vi "速度轉電壓.vi"(1 "Speed (0.1mm/s)":dbl) -> (0 "Voltage\nOutput":dbl)   [LabVIEW 2019]
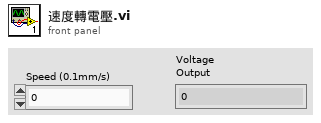
[diagram p1: front panel]
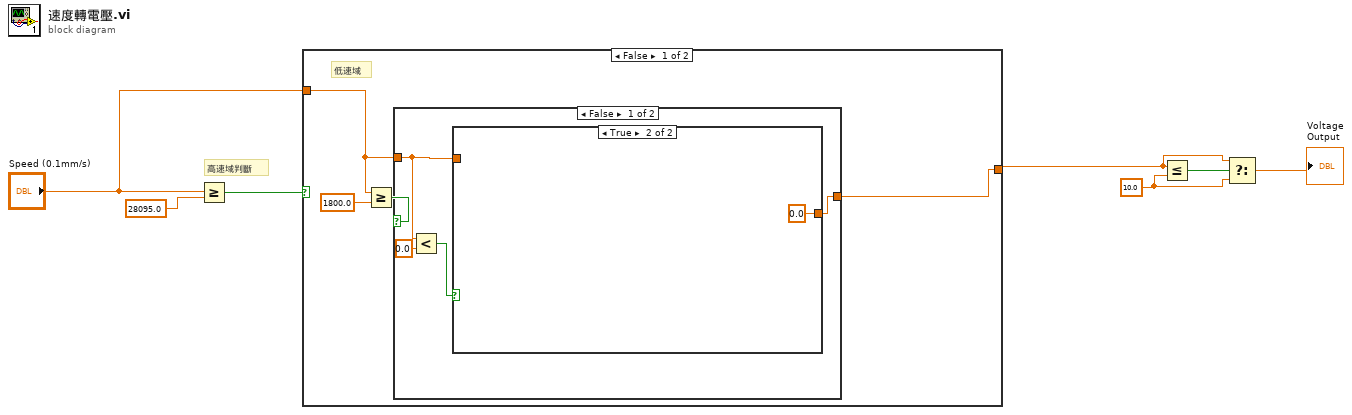
[diagram p0: block diagram]
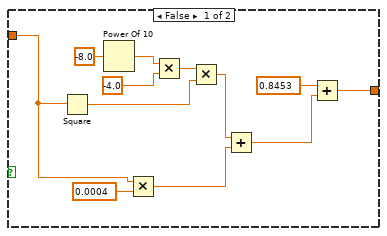
[diagram p2: hidden frame]
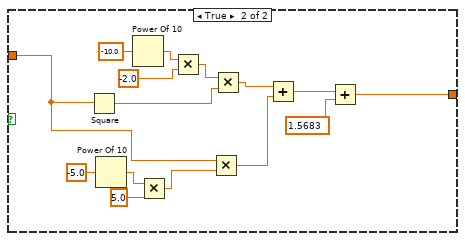
[diagram p3: hidden frame]
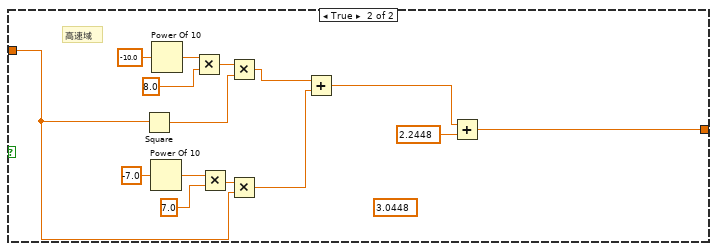
[diagram p4: hidden frame]
diagram:
  w2 = 10.0 ("y")
  # "高速域判斷"
  n1 = Greater Or Equal?(x="Speed (0.1mm/s)", y=28095.0) -> (x >= y?=w6:bool)
  n2 = case shown="False" w6 {
    tunnel: "Speed (0.1mm/s)" -> [w9 w48]
    tunnel: [w8 w58] -> w3
    frame False {
      # "低速域"
      n3 = Greater Or Equal?(x=w9, y=1800.0) -> (x >= y?=w10:bool)
      n4 = case shown="False" w10 {
        tunnel: w9 -> [w13 w34]
        tunnel: [w15 w30] -> w8
        frame False {
          n5 = Less?(x=w13, y=0.0) -> (x < y?=w14:bool)
          n6 = case shown="True" w14 {
            tunnel: [w17 0.0] -> w15
            tunnel: w13 -> [w16 _]
            frame False {
              n7 = Square(x=w16) -> (x^2=w27:dbl)
              n8 = Power Of 10(x=-8.0) -> (10^x=w22:dbl)
              n9 = Multiply(x=w16, y=0.0004) -> (x*y=w24:dbl)
              n10 = Multiply(x=w22, y=-4.0) -> (x*y=w26:dbl)
              n11 = Multiply(x=w26, y=w27) -> (x*y=w25:dbl)
              n12 = Add(x=w25, y=w24) -> (x+y=w23:dbl)
              n13 = Add(x=0.8453, y=w23) -> (x+y=w17:dbl)
            }
            frame True {
            }
          }
        }
        frame True {
          n14 = Square(x=w34) -> (x^2=w39:dbl)
          n15 = Power Of 10(x=-5.0) -> (10^x=w37:dbl)
          n16 = Power Of 10(x=-10.0) -> (10^x=w43:dbl)
          n17 = Multiply(x=w37, y=5.0) -> (x*y=w33:dbl)
          n18 = Multiply(x=w43, y=-2.0) -> (x*y=w40:dbl)
          n19 = Multiply(x=w34, y=w33) -> (x*y=w32:dbl)
          n20 = Multiply(x=w40, y=w39) -> (x*y=w38:dbl)
          n21 = Add(x=w38, y=w32) -> (x+y=w31:dbl)
          n22 = Add(x=w31, y=1.5683) -> (x+y=w30:dbl)
        }
      }
    }
    frame True {
      (unwired) 3.0448 ("y")
      # "高速域"
      n23 = Square(x=w48) -> (x^2=w53:dbl)
      n24 = Power Of 10(x=-7.0) -> (10^x=w51:dbl)
      n25 = Power Of 10(x=-10.0) -> (10^x=w56:dbl)
      n26 = Multiply(x=w56, y=8.0) -> (x*y=w54:dbl)
      n27 = Multiply(x=w51, y=7.0) -> (x*y=w49:dbl)
      n28 = Multiply(x=w54, y=w53) -> (x*y=w47:dbl)
      n29 = Multiply(x=w49, y=w48) -> (x*y=w46:dbl)
      n30 = Add(x=w47, y=w46) -> (x+y=w45:dbl)
      n31 = Add(x=w45, y=2.2448) -> (x+y=w58:dbl)
    }
  }
  n32 = Less Or Equal?(x=w3, y=w2) -> (x <= y?=w4:bool)
  n33 = Select(t=w3, s=w4, f=w2) -> (s? t:f=→"Voltage\nOutput":dbl)
